vi "FSK.vi"() -> ()   [LabVIEW 2023]
uses:
  <vilib>/Analysis/NI_AALPro.lvlib
panel:
  out "Array":bool[](array[boolean])
  out "Waveform Chart":dbl[](graph)
  out "Waveform Chart 2":dbl[](graph)
  in  "signal type":T1(ring)
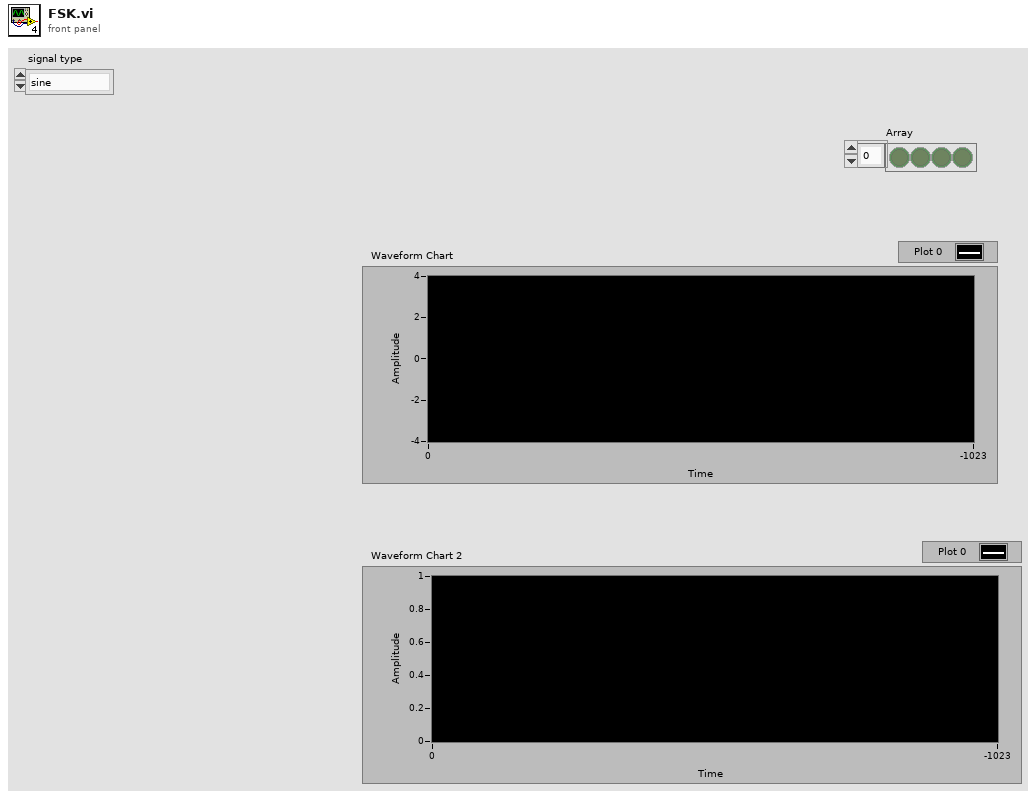
[diagram p1: front panel]
types:
  T1 = enum16{"sine", "cosine", "triangle", "square", "sawtooth", "increasing ramp", "decreasing ramp"}
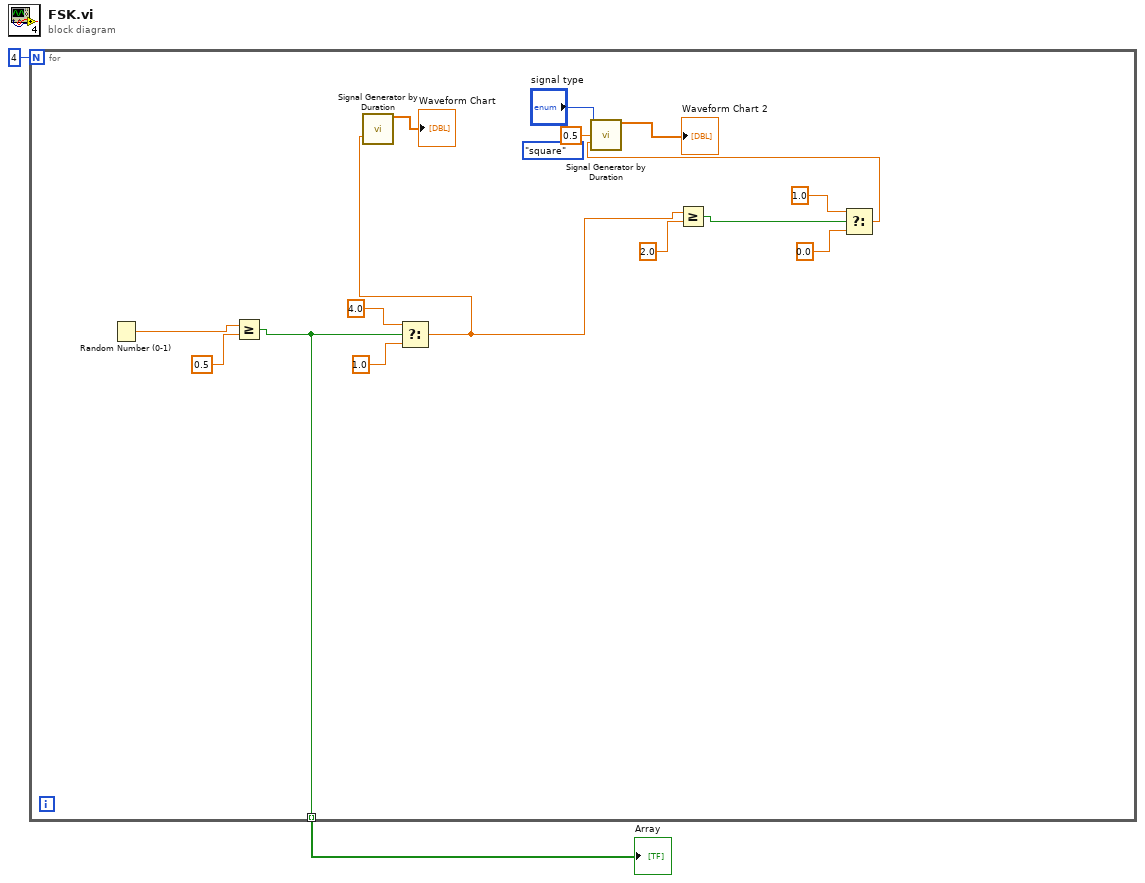
[diagram p0: block diagram]
diagram:
  n1 = for {
    N: 4 -> [_]
    tunnel: [w4] -> w1 mode=indexing
    (unwired) T1."square" ("signal type")
    n2 = Random Number (0-1)() -> (number: 0 to 1=w17:dbl)
    n3 = Greater Or Equal?(x=w17, y=0.5) -> (x >= y?=w4:bool)
    n4 = Select(t=4.0, s=w4, f=1.0) -> (s? t:f=w7:dbl)
    n5 = call <vilib>:"Signal Generator by Duration.vi"("amplitude"=w7) -> ("signal"=→"Waveform Chart":dbl[])  [unwired: 11 in, 3 out]
    n6 = Greater Or Equal?(x=w7, y=2.0) -> (x >= y?=w12:bool)
    n7 = Select(t=1.0, s=w12, f=0.0) -> (s? t:f=w9:dbl)
    n8 = call <vilib>:"Signal Generator by Duration.vi"("signal type"="signal type", "frequency"=0.5, "amplitude"=w9) -> ("signal"=→"Waveform Chart 2":dbl[])  [unwired: 9 in, 3 out]
  }
  "Array" <- w1
